vi "WaveformChart.vi"() -> ()   [LabVIEW 2025]
doc: "Generates random data and plots it dynamically on a waveform chart to visualize real-time changes."
uses:
  <vilib>/numeric/Random Number (Range) DBL.vi
panel:
  in  "lower limit":dbl
  in  "upper limit":dbl
  in  "?":bool
  out "Randon data Chart":dbl(graph)
  # "Sample example of generating random data in waveform chart"
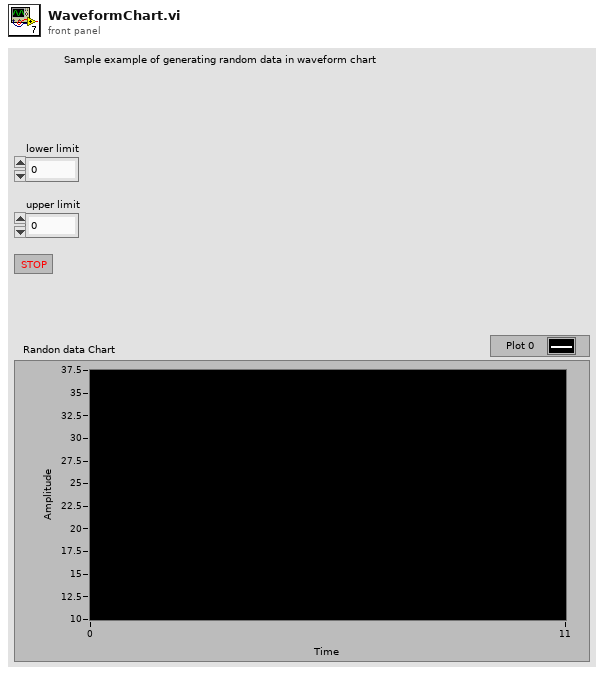
[diagram p1: front panel]
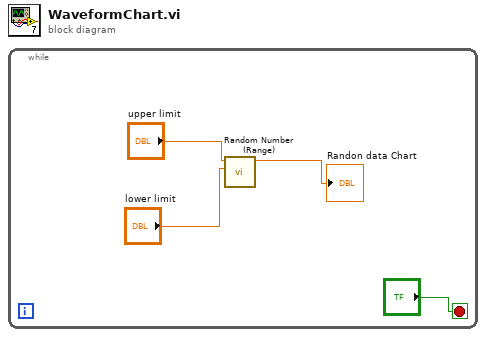
[diagram p0: block diagram]
diagram:
  n1 = while {
    stop <- "?" stop-if-true
    n2 = call-poly <vilib>:"Random Number (Range).vi"("lower bound (0)"="lower limit", "upper bound (100)"="upper limit") -> ("number"=→"Randon data Chart":dbl)  [unwired: 9 in]
  }
